vi "GetTargetBuildSpecs (project reference).vi"(8 "error in (no error)":errorcluster, 9 "Name of target (My Computer)":string="My Computer", 10 "Name of build specification (if empty: get all)":string, 11 "Project reference":refnum<vi>) -> (0 "error out":errorcluster, 2 "buildspec refs":refnum<vi>[](array[refnum]), 3 "project ref":refnum<vi>)   [LabVIEW 2020]
uses:
  <resource>/Framework/Providers/Common/provcom_StringGlobals.vi
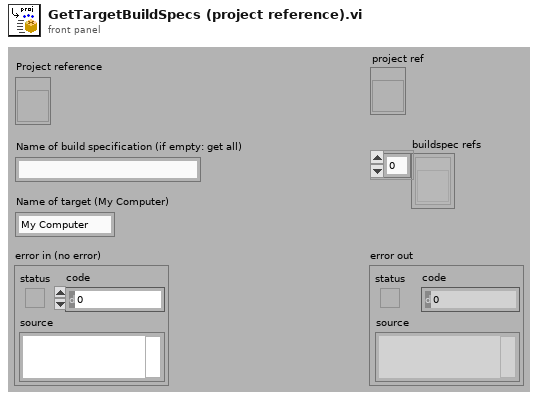
[diagram p1: front panel]
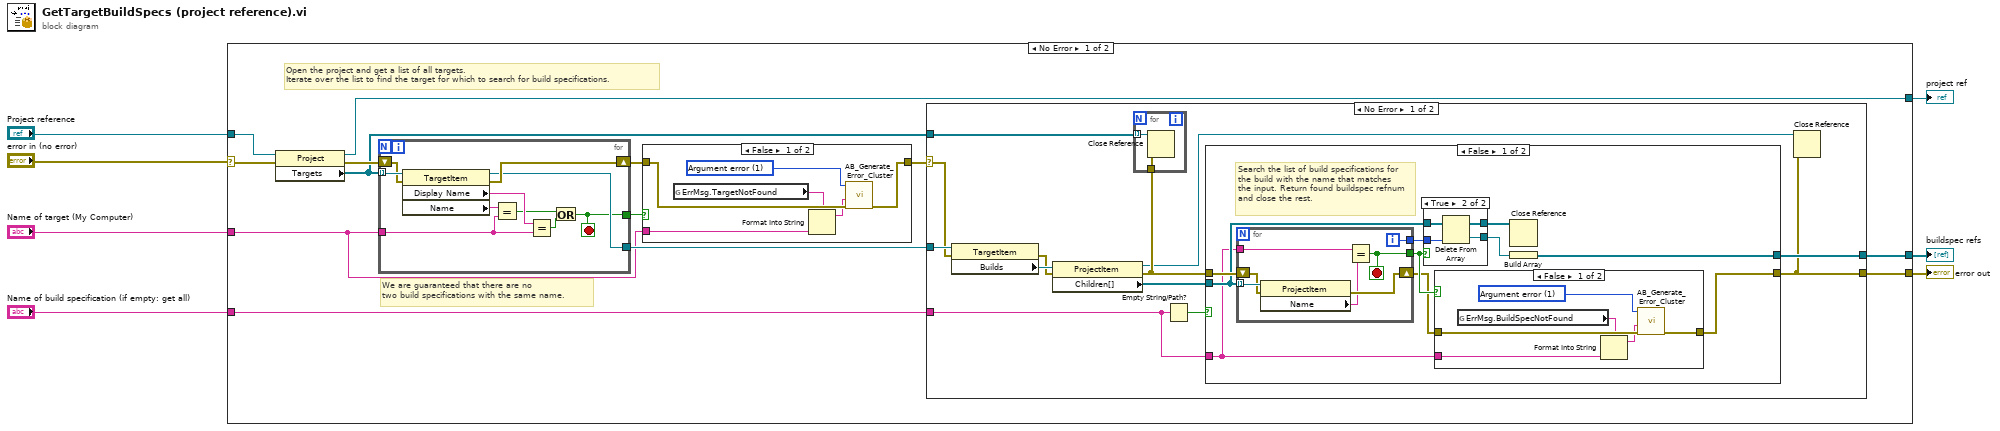
[diagram p0: block diagram]
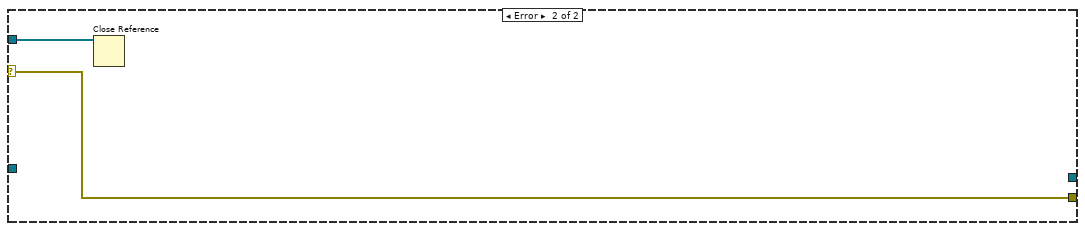
[diagram p6: hidden frame]
diagram:
  n1 = case shown="No Error" "error in (no error)" {
    selector: "error in (no error)" -> [w14 w85]
    tunnel: "Project reference" -> [w15 _]
    tunnel: "Name of target (My Computer)" -> [w8 _]
    tunnel: "Name of build specification (if empty: get all)" -> [w9 _]
    tunnel: [w16 w85] -> w4
    tunnel: [w19 _] -> w1
    tunnel: [w18 _] -> w2
    frame No Error {
      # "We are guaranteed that there are no\ntwo build specifications with the same name."
      # "Open the project and get a list of all targets.\nIterate over the list to find the target for which to search for build specifications."
      n2 = property class="Project"(reference=w15, error in=w14) -> (reference out=w19:refnum<vi>, error out=w20:errorcluster, "Targets"=w17:refnum<vi>[])
      n3 = for {
        tunnel: w17 -> [w84] mode=indexing
        shift-right: [w82] -> w11
        shift-left: w20 -> [w83]
        tunnel: w8 -> [w79]
        tunnel: [w76] -> w13
        tunnel: [w75] -> w12
        stop <- w75 stop-if-true
        n4 = property class="TargetItem"(reference=w84, error in=w83) -> (reference out=w76:refnum<vi>, error out=w82:errorcluster, "Display Name"=w81:string, "Name"=w80:string)
        n5 = Equal?(x=w80, y=w79) -> (x = y?=w78:bool)
        n6 = Equal?(x=w81, y=w79) -> (x = y?=w77:bool)
        n7 = Or(x=w78, y=w77) -> (x .or. y?=w75:bool)
      }
      n8 = case shown="False" w12 {
        tunnel: w11 -> [w26 w27]
        tunnel: [w25 w27] -> w10
        tunnel: w8 -> [w22 _]
        frame False {
          w24 = 1 items=["No error", "Argument error", "Memory is full", "Out of zone", "End of file", "File already open", "Generic file I/O error", "File not found", "File permission error", "Disk is full", "Duplicate path", "Too many files open", "System feature not enabled", "Resource file not found", "Cannot add resource", "Resource not found", "Image not found", "Image memory error", "Pen does not exist", "Config type invalid", "Config token not found", "Config parse error", "Config memory error", "Bad external code format", "Bad external code offset", "External code not present", "Null window", "Destroy window error", "Null menu", "Print aborted", "Bad print record", "Print driver error", "Windows error during printing", "Memory error during printing", "Print dialog error", "Generic print error", "Invalid device refnum", "Device not found", "Device parameter error", "Device unit error", "Cannot open device", "Device call aborted", "Generic error", "Cancelled by user", "Object ID too low", "Object ID too high", "Object not in heap", "Unknown heap", "Unknown object (invalid DefProc)", "Unknown object (DefProc not in table)", "Message out of range", "Invalid (null) method", "Unknown message", "Manager call not supported", "Bad address", "Network operation in progress", "Network operation timed out", "Connection is busy", "Network attribute not supported", "Network error", "Address in use", "System out of memory", "Connection aborted", "Connection refused", "Not connected", "Already connected", "Connection closed", "Initialization error (interapplication manager)", "Bad occurrence", "Wait on unbound occurrence handler", "Occurrence queue overflow", "Datalog type conflict", "Unused", "Unrecognized type (interapplication manager)", "Memory corrupt", "Failed to make temporary DLL", "Old CIN version", "Drag socket not found", "Failed to load drop-object", "Failed to register OLE object", "Failed to release OLE object", "Format specifier type mismatch", "Unknown format specifier", "Too few format specifiers", "Too many format specifiers", "Scan failed", "Newer CIN version", "Error converting to variant", "Runtime menu error", "Password tampered", "Variant attribute not found", "Incompatible variant data type", "Event data is not available", "Event Store is not present", "Occurrence is not found", "Event Queue is not created", "Event info is not available in the type library", "Refnum passed is NULL", "Error retrieving Class GUID", "Error retrieving CoClass GUID", "Error retrieving TypeLib GUID.", "Bad built application magic bytes.", "Specific driver is different from the specific driver associated with the Logical Name.", "There is no session opened to the class driver.", "Max Error", "MAX - Error with config objects", "MAX - Error loading configuration", "MAX - Group not supported", "Singlecast connections can not send to multicast addresses.", "Multicast connections can not send to singlecast addresses.", "Specified IP address not in multicast address range.", "Attempt to write to read-only multicast connection.", "Attempt to read from write-only multicast connection.", "The buffer used to receive a datagram was smaller than the datagram itself"] ("Code")
          n9 = global read "provcom_StringGlobals.vi" "ErrMsg.TargetNotFound"() -> (w23:string)
          n10 = Format Into String(format string=w23, w22) -> (resulting string=w21:string)  [unwired: 2 in, 1 out]
          n11 = call <vilib>:"AB_Generate_Error_Cluster.vi"("error in (no error)"=w26, "Additional Message"=w21, "Code"=w24) -> ("error out"=w25:errorcluster)  [unwired: 1 in, 7 out]
        }
        frame True {
        }
      }
      n12 = case shown="No Error" w10 {
        selector: w10 -> [w28 w74]
        tunnel: w9 -> [w34 _]
        tunnel: [w33 _] -> w18
        tunnel: w17 -> [w32 w73]
        tunnel: [w31 w74] -> w16
        tunnel: w13 -> [w29 _]
        frame No Error {
          n13 = property class="TargetItem"(reference=w29, error in=w28) -> (error out=w38:errorcluster, "Builds"=w39:refnum<vi>)  [unwired: 1 out]
          n14 = property class="ProjectItem"(reference=w39, error in=w38) -> (reference out=w30:refnum<vi>, error out=w37:errorcluster, "Children[]"=w36:refnum<vi>[])
          n15 = for {
            tunnel: w32 -> [w72] mode=indexing
            tunnel: w37 -> [w71]
            n16 = Close Reference(reference=w72, error in (no error)=w71) -> ()  [unwired: 1 out]
          }
          n17 = Empty String/Path?(string/path=w34) -> (empty?=w35:bool)
          n18 = case shown="False" w35 {
            tunnel: w37 -> [w49 w70]
            tunnel: [w41 w70] -> w31
            tunnel: w36 -> [w47 w69]
            tunnel: [w48 w69] -> w33
            tunnel: w34 -> [w40 _]
            frame False {
              # "Search the list of build specifications for the build with the name that matches the input. Return found buildspec refnum and close the rest."
              n19 = for {
                tunnel: w47 -> [w68] mode=indexing
                shift-right: [w66] -> w42
                shift-left: w49 -> [w67]
                tunnel: w40 -> [w62]
                tunnel: [w65] -> w46
                tunnel: [w64] -> w43
                i -> [w65]
                stop <- w64 stop-if-true
                n20 = property class="ProjectItem"(reference=w68, error in=w67) -> (error out=w66:errorcluster, "Name"=w63:string)  [unwired: 1 out]
                n21 = Equal?(x=w62, y=w63) -> (x = y?=w64:bool)
              }
              n22 = case shown="True" w43 {
                tunnel: w47 -> [w57 w61]
                tunnel: w46 -> [_ w60]
                tunnel: [w57 w59] -> w45
                tunnel: [_ w58] -> w44
                frame False {
                }
                frame True {
                  n23 = Delete From Array(array=w61, index=w60) -> (deleted portion=w58:refnum<vi>, array with subset deleted=w59:refnum<vi>[])  [unwired: 1 in]
                }
              }
              n24 = case shown="False" w43 {
                tunnel: w42 -> [w55 w56]
                tunnel: [w54 w56] -> w41
                tunnel: w40 -> [w51 _]
                frame False {
                  w53 = 1 items=["No error", "Argument error", "Memory is full", "Out of zone", "End of file", "File already open", "Generic file I/O error", "File not found", "File permission error", "Disk is full", "Duplicate path", "Too many files open", "System feature not enabled", "Resource file not found", "Cannot add resource", "Resource not found", "Image not found", "Image memory error", "Pen does not exist", "Config type invalid", "Config token not found", "Config parse error", "Config memory error", "Bad external code format", "Bad external code offset", "External code not present", "Null window", "Destroy window error", "Null menu", "Print aborted", "Bad print record", "Print driver error", "Windows error during printing", "Memory error during printing", "Print dialog error", "Generic print error", "Invalid device refnum", "Device not found", "Device parameter error", "Device unit error", "Cannot open device", "Device call aborted", "Generic error", "Cancelled by user", "Object ID too low", "Object ID too high", "Object not in heap", "Unknown heap", "Unknown object (invalid DefProc)", "Unknown object (DefProc not in table)", "Message out of range", "Invalid (null) method", "Unknown message", "Manager call not supported", "Bad address", "Network operation in progress", "Network operation timed out", "Connection is busy", "Network attribute not supported", "Network error", "Address in use", "System out of memory", "Connection aborted", "Connection refused", "Not connected", "Already connected", "Connection closed", "Initialization error (interapplication manager)", "Bad occurrence", "Wait on unbound occurrence handler", "Occurrence queue overflow", "Datalog type conflict", "Unused", "Unrecognized type (interapplication manager)", "Memory corrupt", "Failed to make temporary DLL", "Old CIN version", "Drag socket not found", "Failed to load drop-object", "Failed to register OLE object", "Failed to release OLE object", "Format specifier type mismatch", "Unknown format specifier", "Too few format specifiers", "Too many format specifiers", "Scan failed", "Newer CIN version", "Error converting to variant", "Runtime menu error", "Password tampered", "Variant attribute not found", "Incompatible variant data type", "Event data is not available", "Event Store is not present", "Occurrence is not found", "Event Queue is not created", "Event info is not available in the type library", "Refnum passed is NULL", "Error retrieving Class GUID", "Error retrieving CoClass GUID", "Error retrieving TypeLib GUID.", "Bad built application magic bytes.", "Specific driver is different from the specific driver associated with the Logical Name.", "There is no session opened to the class driver.", "Max Error", "MAX - Error with config objects", "MAX - Error loading configuration", "MAX - Group not supported", "Singlecast connections can not send to multicast addresses.", "Multicast connections can not send to singlecast addresses.", "Specified IP address not in multicast address range.", "Attempt to write to read-only multicast connection.", "Attempt to read from write-only multicast connection.", "The buffer used to receive a datagram was smaller than the datagram itself"] ("Code")
                  n25 = global read "provcom_StringGlobals.vi" "ErrMsg.BuildSpecNotFound"() -> (w52:string)
                  n26 = Format Into String(format string=w52, w51) -> (resulting string=w50:string)  [unwired: 2 in, 1 out]
                  n27 = call <vilib>:"AB_Generate_Error_Cluster.vi"("error in (no error)"=w55, "Additional Message"=w50, "Code"=w53) -> ("error out"=w54:errorcluster)  [unwired: 1 in, 7 out]
                }
                frame True {
                }
              }
              n28 = Close Reference(reference=w45) -> ()  [unwired: 1 in, 1 out]
              n29 = Build Array(w44) -> (w48:refnum<vi>[])
            }
            frame True {
              # "In the empty case, build all of the build specifications under the specified target, in order."
            }
          }
          n30 = Close Reference(reference=w30, error in (no error)=w31) -> ()  [unwired: 1 out]
        }
        frame Error {
          n31 = Close Reference(reference=w73) -> ()  [unwired: 1 in, 1 out]
        }
      }
    }
    frame Error {
    }
  }
  "error out" <- w4
  "buildspec refs" <- w2
  "project ref" <- w1
